vi "filter_frequency_imp_test_v10.vi"() -> ()   [LabVIEW 2014]
uses:
  <vilib>/rvi/Analysis/host/Butterworth/config/Butterworth Filter Order.ctl
  <vilib>/rvi/Analysis/host/Butterworth/config/Butterworth Filter Type.ctl
  <vilib>/FPGAPlugInAG/cRIO-9039/niLvFpga_Open_cRIO-9039.vi
  <vilib>/rvi/interface/common/dynamic/niFpgaDynamicAddResources.vi
  <vilib>/rvi/Analysis/host/Butterworth/config/BwScaledCoefficients.vi
  <vilib>/Utility/error.llb/Error Cluster From Error Code.vi
  <vilib>/rvi/errors/niLvFpgaAdjustHostInterfaceError.vi
  <vilib>/FPGAPlugInAG/Dynamic/niLvFpga_Close_Dynamic.vi
  <vilib>/rvi/interface/nirviOpenFPGA/nirviOpenFPGA.xnode
  FPGA Bitfiles/test0304_FPGATarget_imptestv102_ot3i2MNL5CE.lvbitx
  FPGA VIs/imp_test_v10_2.vi
  <vilib>/rvi/Analysis/host/Butterworth/XNode/ButterworthCoefficients.xnode
  <vilib>/rvi/interface/nirviReadWriteControl/nirviReadWriteControl.xnode
  <vilib>/rvi/interface/nirviCloseFPGA/nirviCloseFPGA.xnode
  <vilib>/rvi/Analysis/host/Public/NI_FpgaMspHost.lvlib
  NiFpgaLv.dll
  <vilib>/rvi/interface/Simulation/niFpgaSimulationCallBeginRW.vi
panel:
  in  "sr_omega_y_Mavg (S/s)":dbl=50000.0
  in  "fcu_omega_y_Mavg (Hz)":dbl=1000.0
  in  "sr_omega_p_Mavg (S/s)":dbl=50000.0
  in  "fcu_omega_p_Mavg (Hz)":dbl=1000.0
  in  "Filter set":bool
  in  "sr_Strain(Avg.8)_p (S/s)":dbl=50000.0
  in  "fcu_Strain(Avg.8)_p (Hz)":dbl=1000.0
  in  "sr_Dp_dd (S/s)":dbl=50000.0
  in  "fcu_Dp_dd (Hz)":dbl=1000.0
  in  "sr_dFp_PIS (S/s)":dbl=50000.0
  in  "fcu_dFp_PID (Hz)":dbl=1000.0
  in  "sr_Strain(Avg.8)_y (S/s)":dbl=50000.0
  in  "fcu_Strain(Avg.8)_y (Hz)":dbl=1000.0
  in  "sr_Dy_dd (S/s)":dbl=50000.0
  in  "fcu_Dy_dd (Hz)":dbl=1000.0
  in  "sr_dFy_PID (S/s)":dbl=50000.0
  in  "fcu_dFy_PID (Hz)":dbl=1000.0
  in  "stop":bool
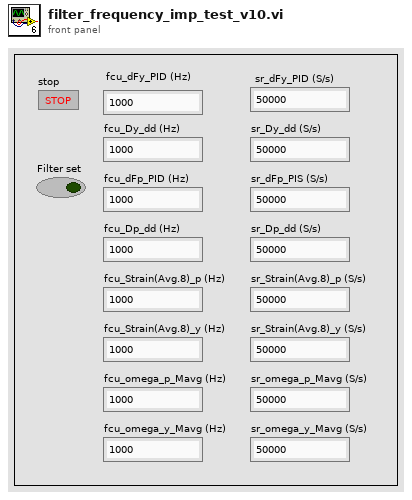
[diagram p1: front panel]
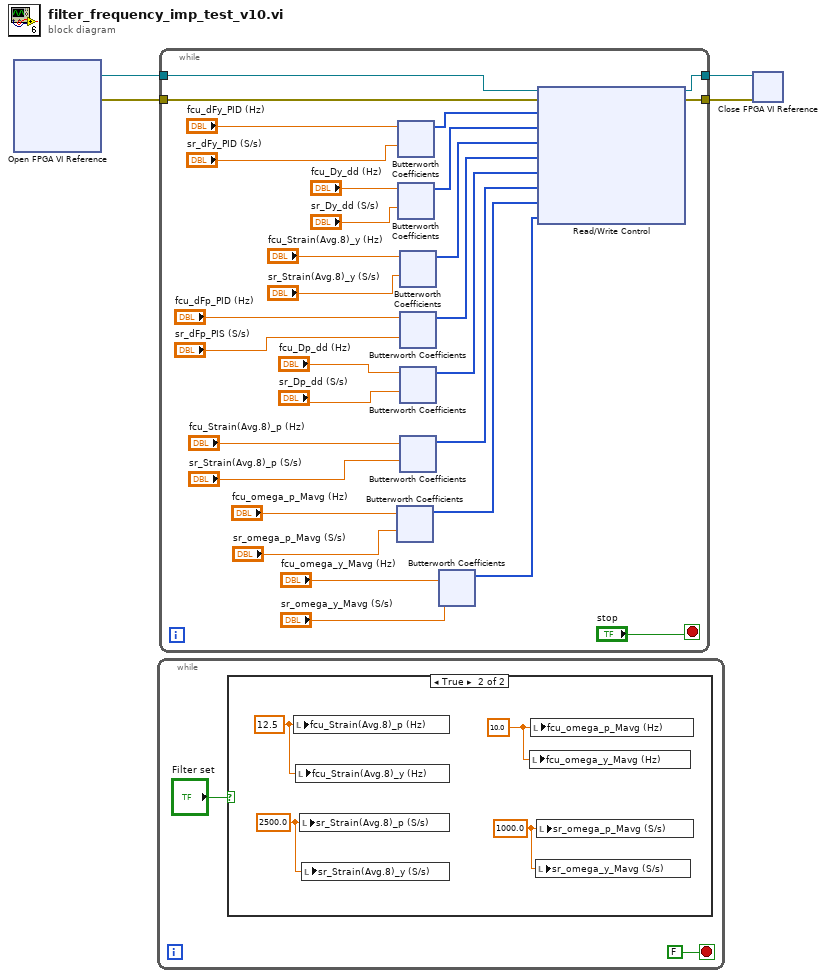
[diagram p0: block diagram]
diagram:
  n1 = xnode "Open FPGA VI Reference"() -> ("FPGA VI Reference Out"=w4:refnum<k20>, "error out"=w3:errorcluster)  [unwired: 2 in]
  n2 = while {
    stop <- FALSE stop-if-true
    n3 = case shown="True" "Filter set" {
      frame False {
      }
      frame True {
        w7 = 1000.0 ("sr_omega_p_Mavg (S/s)")
        w8 = 10.0 ("fcu_omega_p_Mavg (Hz)")
        w9 = 2500.0 ("sr_Strain(Avg.8)_p (S/s)")
        w10 = 12.5 ("fcu_Strain(Avg.8)_p (Hz)")
        n4 = local write "fcu_Strain(Avg.8)_p (Hz)"(w10) -> ()
        n5 = local write "fcu_Strain(Avg.8)_y (Hz)"(w10) -> ()
        n6 = local write "sr_Strain(Avg.8)_p (S/s)"(w9) -> ()
        n7 = local write "sr_Strain(Avg.8)_y (S/s)"(w9) -> ()
        n8 = local write "fcu_omega_y_Mavg (Hz)"(w8) -> ()
        n9 = local write "fcu_omega_p_Mavg (Hz)"(w8) -> ()
        n10 = local write "sr_omega_y_Mavg (S/s)"(w7) -> ()
        n11 = local write "sr_omega_p_Mavg (S/s)"(w7) -> ()
      }
    }
  }
  n12 = while {
    tunnel: w4 -> [w30]
    tunnel: w3 -> [w39]
    tunnel: [w38] -> w2
    tunnel: [w37] -> w1
    stop <- "stop" stop-if-true
    n13 = xnode "Butterworth Coefficients"("cutoff frequency (Hz)"="fcu_omega_p_Mavg (Hz)", "sample rate (S/s)"="sr_omega_p_Mavg (S/s)") -> ("scaled coefficients"=w16:i32[])  [unwired: 1 in, 1 out]
    n14 = xnode "Butterworth Coefficients"("cutoff frequency (Hz)"="fcu_dFy_PID (Hz)", "sample rate (S/s)"="sr_dFy_PID (S/s)") -> ("scaled coefficients"=w29:i32[])  [unwired: 1 in, 1 out]
    n15 = xnode "Butterworth Coefficients"("cutoff frequency (Hz)"="fcu_Dy_dd (Hz)", "sample rate (S/s)"="sr_Dy_dd (S/s)") -> ("scaled coefficients"=w28:i32[])  [unwired: 1 in, 1 out]
    n16 = xnode "Butterworth Coefficients"("cutoff frequency (Hz)"="fcu_Strain(Avg.8)_y (Hz)", "sample rate (S/s)"="sr_Strain(Avg.8)_y (S/s)") -> ("scaled coefficients"=w27:i32[])  [unwired: 1 in, 1 out]
    n17 = xnode "Butterworth Coefficients"("cutoff frequency (Hz)"="fcu_dFp_PID (Hz)", "sample rate (S/s)"="sr_dFp_PIS (S/s)") -> ("scaled coefficients"=w26:i32[])  [unwired: 1 in, 1 out]
    n18 = xnode "Butterworth Coefficients"("cutoff frequency (Hz)"="fcu_Dp_dd (Hz)", "sample rate (S/s)"="sr_Dp_dd (S/s)") -> ("scaled coefficients"=w25:i32[])  [unwired: 1 in, 1 out]
    n19 = xnode "Butterworth Coefficients"("cutoff frequency (Hz)"="fcu_Strain(Avg.8)_p (Hz)", "sample rate (S/s)"="sr_Strain(Avg.8)_p (S/s)") -> ("scaled coefficients"=w18:i32[])  [unwired: 1 in, 1 out]
    n20 = xnode "Butterworth Coefficients"("cutoff frequency (Hz)"="fcu_omega_y_Mavg (Hz)", "sample rate (S/s)"="sr_omega_y_Mavg (S/s)") -> ("scaled coefficients"=w13:i32[])  [unwired: 1 in, 1 out]
    n21 = xnode "Read/Write Control"("FPGA VI Reference In"=w30, "error in"=w39, "dFy_PID coeff."=w29, "Dy_dd coeff."=w28, "Strain_y Avg8 coeff."=w27, "dFp_PID coeff."=w26, "Dp_dd coeff."=w25, "Strain_p Avg.8 coeff."=w18, "omega_P(Mavg) coeff."=w16, "omega_y(Mavg) coeff."=w13) -> ("FPGA VI Reference Out"=w38:refnum<k20>, "error out"=w37:errorcluster)
  }
  n22 = xnode "Close FPGA VI Reference"("FPGA VI Reference In"=w2, "error in"=w1) -> ()  [unwired: 1 out]
